vi "ChangeEccentricity.vi"(7 "Steps":i32, 8 "Time":dbl, 9 "e_f":dbl, 10 "e_0":dbl, 11 "Cluster in":T1 {"Eccentricity" min=0.0; "Size" step=1; "LatC" step=0.05}) -> (3 "Cluster out":T1 {"Eccentricity" min=0.0; "Size" step=1; "LatC" step=0.05})   [LabVIEW 2017]
uses:
  Drawing/CircleControls.ctl
  AODControl/AODGlobals.vi
  AODControl/MessageQueue/QueueOperations/Enqueue Message (Single).vi
  AODControl/MessageQueue/MessageQueue.lvlib
  AODControl/AODControl.lvlib
panel:
  out "Radius":dbl
  out "Eccentricity":dbl
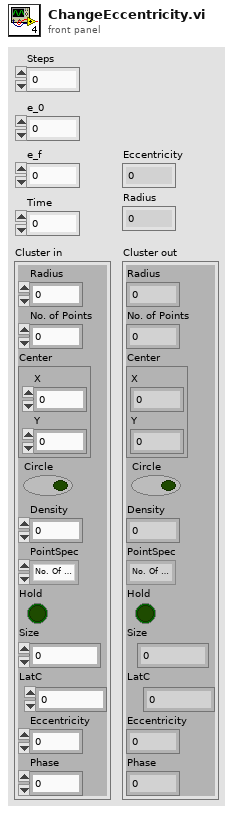
[diagram p1: front panel]
types:
  T1 = typedef "CircleControls.ctl" = cluster{"Radius":dbl, "No. of Points":i32, "Center":cluster{"X":dbl, "Y":dbl}, "Circle":bool, "Density":dbl, "PointSpec":enum32{"No. Of Points", "Density"}, "Hold":bool, "Size":i32, "LatC":dbl, "Eccentricity":dbl, "Phase":dbl}
  T2 = typedef "AODControl.lvlib/MessageQueue.lvlib/All Message Queues.ctl" = cluster{" AOD Interface":refnum<queue>}
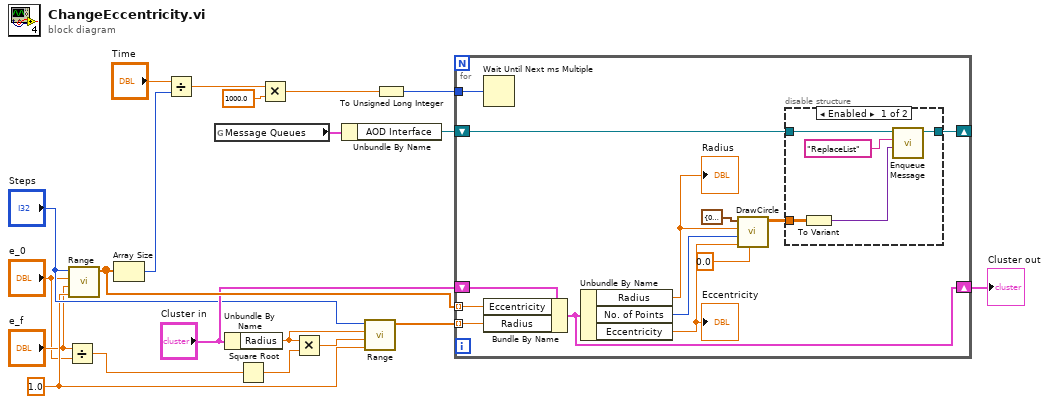
[diagram p0: block diagram]
diagram:
  w8 = 1.0 ("Exponent")
  n1 = Divide(x="e_f", y="e_0") -> (x/y=w5:dbl)
  n2 = call "Range.vi"("Exponent"=w8, "End"="e_f", "Start"="e_0", "Steps"="Steps") -> ("Array"=w11:dbl[])  [unwired: 7 in]
  n3 = Array Size(array=w11) -> (size(s)=w17:i32)
  n4 = Divide(x="Time", y=w17) -> (x/y=w15:dbl)
  n5 = global read "AODGlobals.vi" "Message Queues"() -> (w19:T2)
  n6 = Unbundle By Name("Cluster in") -> ("Radius"=w3:dbl)
  n7 = Square Root(x=w5) -> (sqrt(x)=w4:dbl)
  n8 = Multiply(x=w15, y=1000.0) -> (x*y=w13:dbl)
  n9 = Multiply(x=w3, y=w4) -> (x*y=w2:dbl)
  n10 = Unbundle By Name(w19) -> ("AOD Interface"=w18:refnum<queue>)
  n11 = call "Range.vi"("Exponent"=w8, "End"=w2, "Start"=w3, "Steps"="Steps") -> ("Array"=w1:dbl[])  [unwired: 7 in]
  n12 = To Unsigned Long Integer(number=w13) -> (unsigned 32bit integer=w12:u32)
  n13 = for {
    tunnel: w11 -> [w33] mode=indexing
    shift-right: [w25] -> _
    shift-left: w18 -> [w24]
    tunnel: w12 -> [w22]
    shift-right: [w26] -> w20
    shift-left: "Cluster in" -> [w32]
    tunnel: w1 -> [w21] mode=indexing
    n14 = Wait Until Next ms Multiple(millisecond multiple=w22) -> ()  [unwired: 1 out]
    n15 = Bundle By Name(cluster=w32, "Eccentricity"=w33, "Radius"=w21) -> (w26:T1)
    n16 = Unbundle By Name(w26) -> ("Radius"=w29:dbl, "No. of Points"=w30:i32, "Eccentricity"=w31:dbl)
    "Eccentricity" <- w31
    "Radius" <- w29
    n17 = call "DrawCircle.vi"("Phase"=0.0, "Eccentricity"=w31, "No Of Points"=w30, "Radius"=w29, "Center"=cluster{"X":dbl, "Y":dbl} {"X"=0.0, "Y"=0.0}) -> ("Array"=w23:dbl[][])  [unwired: 6 in]
    n18 = disable-structure shown="Enabled" {
      disable-tunnel: w23 -> [w36 _]
      disable-tunnel: [w35 w39] -> w25
      disable-tunnel: w24 -> [w34 w39]
      frame Enabled {
        n19 = To Variant(anything=w36) -> (Variant=w37:variant)
        n20 = call-poly "Enqueue Message.vi"("Message Data"=w37, "Message"="ReplaceList", "Message Queue"=w34) -> ("dup Message Queue"=w35:refnum<queue>)  [unwired: 7 in, 1 out]
      }
      frame Disabled {
      }
    }
  }
  "Cluster out" <- w20
